vi "Check Iteration Numbers.vi"(8 "error in (no error)":errorcluster, 9 "Channel Name":string="Iteration", 10 "Group Name":string, 11 "Refnum in":refnum<k34>) -> (0 "error out":errorcluster, 2 "Passed ?":bool, 3 "Refnum out":refnum<k34>)   [LabVIEW 2026, in "Telemetry System Tests.lvclass"]
uses:
  Telemetry System Tests.lvclass
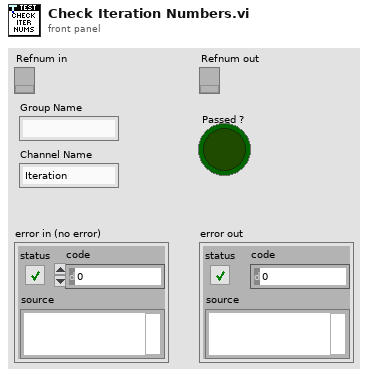
[diagram p1: front panel]
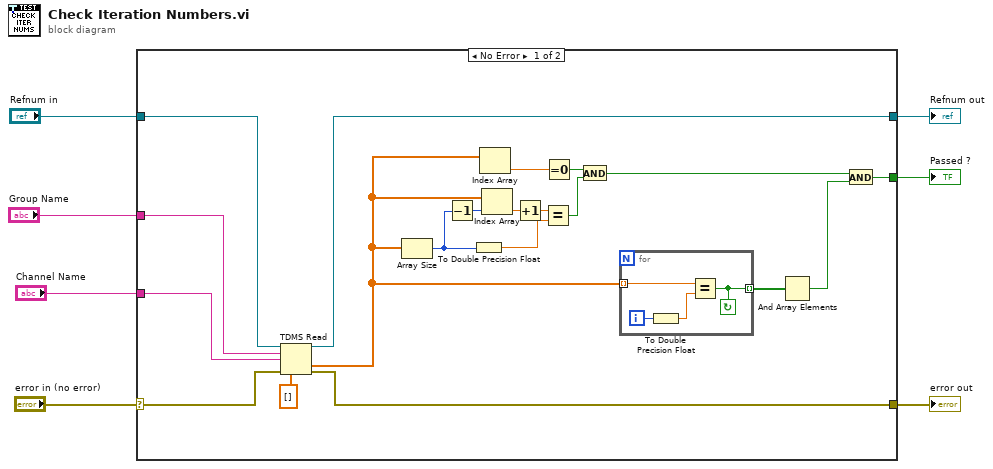
[diagram p0: block diagram]
diagram:
  n1 = case shown="No Error" "error in (no error)" {
    selector: "error in (no error)" -> [w10 w32]
    tunnel: [w17 w33] -> w7
    tunnel: [w16 w32] -> w6
    tunnel: "Refnum in" -> [w14 w33]
    tunnel: [w11 _] -> w4
    tunnel: "Group Name" -> [w9 _]
    tunnel: "Channel Name" -> [w8 _]
    frame No Error {
      n2 = TDMS Read(0:w14, 5:w9, 7:w8, 11:w10, 12:dbl[] []) -> (4:w17:refnum<k34>, 10:w26:dbl[], 15:w16:errorcluster)  [unwired: 3 in, 3 out]
      n3 = Array Size(array=w26) -> (size(s)=w19:i32)
      n4 = Decrement(x=w19) -> (x-1=w18:i32)
      n5 = To Double Precision Float(number=w19) -> (double precision float=w20:dbl)
      n6 = Index Array(array=w26) -> (element=w23:dbl)  [unwired: 1 in]
      n7 = Index Array(array=w26, index=w18) -> (element=w21:dbl)
      n8 = Increment(x=w21) -> (x+1=w22:dbl)
      n9 = Equal?(x=w22, y=w20) -> (x = y?=w25:bool)
      n10 = Equal To 0?(x=w23) -> (x = 0?=w24:bool)
      n11 = And(x=w24, y=w25) -> (x .and. y?=w12:bool)
      n12 = for {
        tunnel: w26 -> [w29] mode=indexing
        tunnel: [w28] -> w27 mode=indexing
        i -> [w31]
        stop <- w28 continue-if-true
        n13 = To Double Precision Float(number=w31) -> (double precision float=w30:dbl)
        n14 = Equal?(x=w29, y=w30) -> (x = y?=w28:bool)
      }
      n15 = And Array Elements(Boolean array=w27) -> (logical AND=w13:bool)
      n16 = And(x=w12, y=w13) -> (x .and. y?=w11:bool)
    }
    frame Error {
    }
  }
  "Refnum out" <- w7
  "error out" <- w6
  "Passed ?" <- w4
